vi "write binary file advanced.vi"() -> ()   [LabVIEW 2016]
uses:
  <vilib>/measure/NI_MABase.lvlib
panel:
  out "Array":dbl[](array[numeric])
  out "Selected Path":path
  out "Data to file":waveform(dbl)(graph)
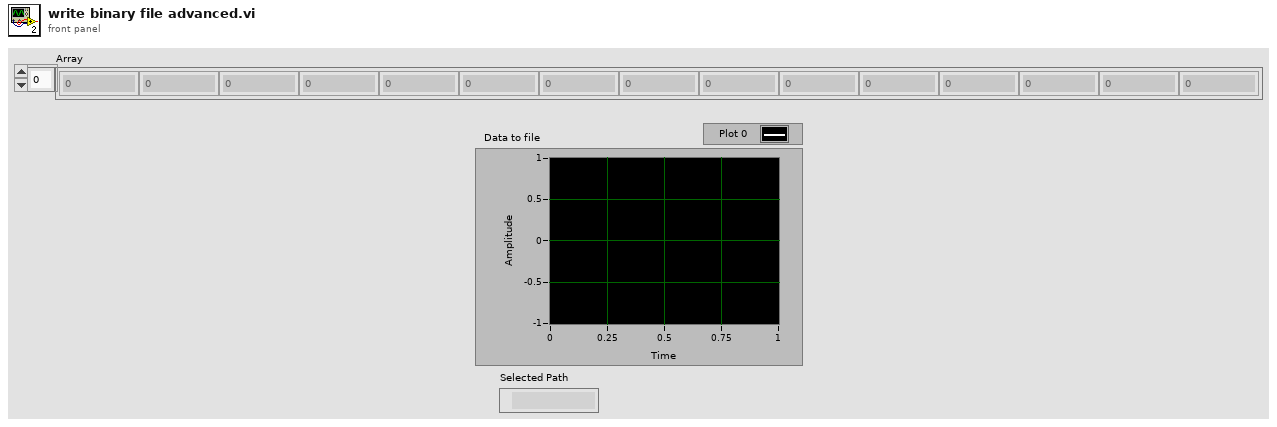
[diagram p1: front panel]
types:
  T1 = enum16{"big-endian, network order", "native, host order", "little-endian"}
  T2 = enum16{"open", "replace", "create", "open or create", "replace or create", "replace or create with confirmation"}
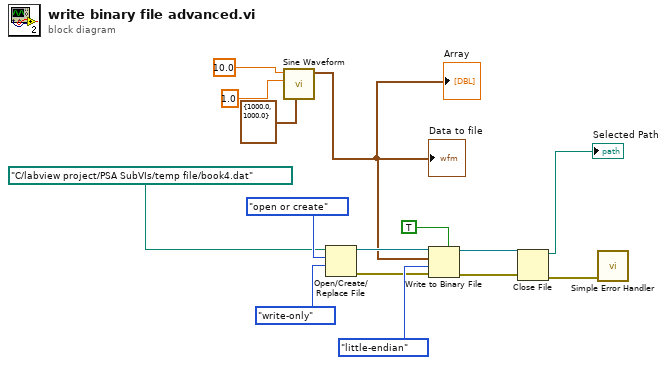
[diagram p0: block diagram]
diagram:
  n1 = call <vilib>:"Sine Waveform.vi"("sampling info"=cluster{"Fs":dbl, "#s":dbl} {"Fs"=1000.0, "#s"=1000.0}, "amplitude"=1.0, "frequency"=10.0) -> ("signal out"=w1:waveform(dbl))  [unwired: 7 in, 1 out]
  "Data to file" <- w1
  "Array" <- w1
  n2 = Open/Create/Replace File(file path (use dialog)=path "C:/labview project/PSA SubVIs/temp file/book4.dat", operation (0:open)=T2."open or create", access (0:read/write)=enum16{"read/write", "read-only", "write-only"}."write-only") -> (refnum out=w11:refnum<file>, error out=w7:errorcluster)  [unwired: 3 in, 1 out]
  n3 = Write to Binary File(file (use dialog)=w11, data=w1, error in=w7, 5:TRUE ("prepend array or string size? (T)"), 9:T1."little-endian" ("byte order (0:big-endian, network order)")) -> (refnum out=w9:refnum<file>, error out=w8:errorcluster)  [unwired: 1 in, 1 out]
  n4 = Close File(refnum=w9, error in=w8) -> (path=→"Selected Path":path, error out=w5:errorcluster)
  n5 = call <vilib>:"Simple Error Handler.vi"("error in (no error)"=w5) -> ()  [unwired: 4 in, 5 out]
